vi "Get Object to File (Sequential).vi"(6 "Version ID":string, 7 "Chunk size (kB)":i32=1024 min=1024, 8 "error in (no error)":errorcluster, 9 "Bucket":string, 10 "Object Path":string, 11 "File path":path) -> (0 "error out":errorcluster)   [LabVIEW 2011, in "LV Interface for Amazon S3.lvlib"]
doc: "This operation <B>retrieves an object</B> from Amazon S3 <B>to a file</B>. The operation <B>retrieves object data in chunks</B>. You <B>must have READ access</B> to the object. If you grant READ access to the anonymous user, you can return the object without using an authorization header. To distribute large files to many people, you can <B>save bandwidth costs using BitTorrent</B>."
uses:
  LV Interface for Amazon S3.lvlib
  Typedefs/AMZ_S3_API_GET Object Request Parameters.ctl
  Typedefs/AMZ_S3_API_GET Request Range.ctl
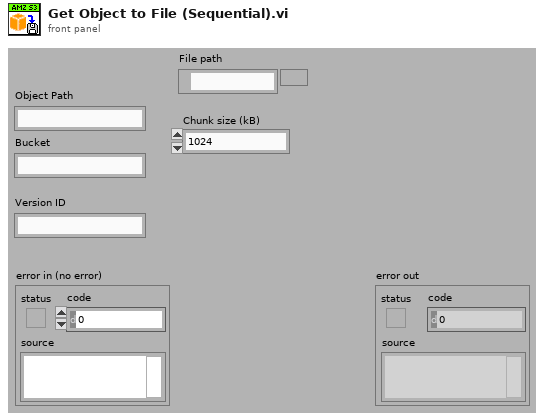
[diagram p1: front panel]
types:
  T1 = enum16{"open", "replace", "create", "open or create", "replace or create", "replace or create with confirmation"}
  T2 = typedef "LV Interface for Amazon S3.lvlib/AMZ_S3_API_GET Object Request Parameters.ctl" = cluster{"Range":T3, "If Modified Since":timestamp, "If Unmodified Since":timestamp, "Matching ETag":string, "Nonmatching ETag":string}
  T3 = typedef "LV Interface for Amazon S3.lvlib/AMZ_S3_API_GET Request Range.ctl" = cluster{"Start":i64, "Length":i64}
  T4 = typedef "LV Interface for Amazon S3.lvlib/AMZ_S3_API_GETObjectResult.ctl" = cluster{"Content Length (bytes)":u64, "Content Type":string, "ETag":string, "Delete marker":bool, "Version ID":string, "Object Size (bytes)":u64}
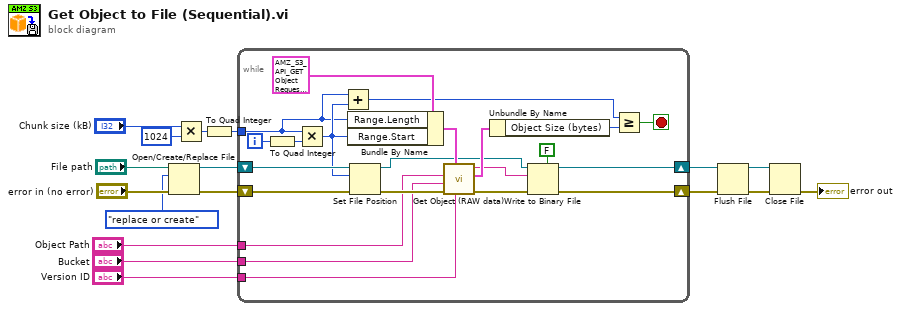
[diagram p0: block diagram]
diagram:
  n1 = Open/Create/Replace File(file path (use dialog)="File path", error in="error in (no error)", operation (0:open)=T1."replace or create") -> (refnum out=w14:refnum<file>, error out=w13:errorcluster)  [unwired: 3 in, 1 out]
  n2 = Multiply(x="Chunk size (kB)", y=1024) -> (x*y=w2:i32)
  n3 = To Quad Integer(1:w2) -> (0:w1:i64)
  n4 = while {
    tunnel: w1 -> [w18]
    tunnel: "Object Path" -> [w29]
    tunnel: "Bucket" -> [w28]
    shift-right: [w23] -> w9
    shift-left: w14 -> [w32]
    shift-right: [w24] -> w10
    shift-left: w13 -> [w33]
    tunnel: "Version ID" -> [w22]
    i -> [w20]
    stop <- w34 stop-if-true
    n5 = To Quad Integer(1:w20) -> (0:w19:i64)
    n6 = Multiply(x=w18, y=w19) -> (x*y=w31:i64)
    n7 = Add(x=w18, y=w31) -> (x+y=w35:i64)
    n8 = Bundle By Name(cluster=T2 {"Range"={"Start"=0, "Length"=0}, "If Modified Since"=timestamp(0 s since 1904-01-01), "If Unmodified Since"=timestamp(0 s since 1904-01-01), "Matching ETag"="", "Nonmatching ETag"=""} ("Request Parameters"), "Range.Length"=w18, "Range.Start"=w31) -> (w38:T2)
    n9 = Set File Position(offset (in bytes) (0)=w31, refnum=w32, error in=w33) -> (refnum out=w25:refnum<file>, error out=w30:errorcluster)  [unwired: 1 in]
    n10 = call "Get Object (RAW data).vi"("Version ID"=w22, "Request Parameters"=w38, "error in (no error)"=w30, "Bucket"=w28, "Path"=w29) -> ("error out"=w27:errorcluster, "GetObjectResult"=w37:T4, "Data"=w26:string)  [unwired: 4 in]
    n11 = Unbundle By Name(w37) -> ("Object Size (bytes)"=w36:u64)
    n12 = Write to Binary File(file (use dialog)=w25, data=w26, error in=w27, 5:FALSE ("prepend array or string size? (T)")) -> (refnum out=w23:refnum<file>, error out=w24:errorcluster)  [unwired: 2 in, 1 out]
    n13 = Greater Or Equal?(x=w35, y=w36) -> (x >= y?=w34:bool)
  }
  n14 = Flush File(refnum=w9, error in=w10) -> (refnum out=w7:refnum<file>, error out=w8:errorcluster)
  n15 = Close File(refnum=w7, error in=w8) -> (error out=→"error out":errorcluster)  [unwired: 1 out]
